vi "Display Required Helper.vi"(8 "Display Required Argument":T2, 11 "Module Data":T3) -> (0 "Display Required (Reply Payload)":T1, 1 "Message":string, 3 "Module Data out":T3)   [LabVIEW 2024, in "DQMH Power Requests.lvlib"]
doc: "<b>Note:</b> This VI was modified by the <b>Validate DQMH Module</b> tool to turn off automatic error handling.\n\n<b>Note:</b> This VI was modified by the <b>Validate DQMH Module</b> tool to be shared clone reentrant."
uses:
  DQMH Power Requests.lvlib
  Module Data--cluster.ctl
  Display Required Argument--cluster.ctl
  Display Required (Reply Payload)--cluster.ctl
  Power-Requests/Power Availabilty Requests/Type Defs/Power Availiability Requests Functions.ctl
  Power-Requests/Power Availabilty Requests/Type Defs/Power Request Type.ctl
  <vilib>/Utility/error.llb/Error Cluster From Error Code.vi
  <vilib>/ErrorRing/Error Ring.xnode
  Power-Requests/Power Requests.lvlib
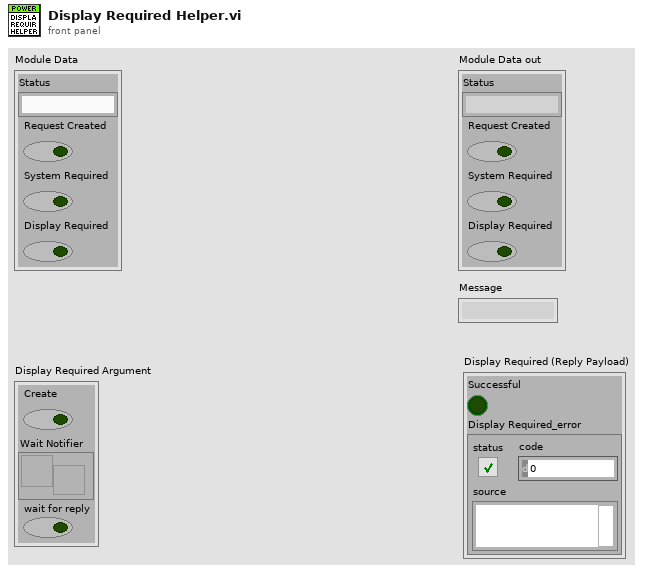
[diagram p1: front panel]
types:
  T1 = typedef "DQMH Power Requests.lvlib/Display Required (Reply Payload)--cluster.ctl" = cluster{"Successful":bool, "Display Required_error":errorcluster}
  T2 = typedef "DQMH Power Requests.lvlib/Display Required Argument--cluster.ctl" = cluster{"Create":bool, "Wait Notifier":refnum<notifier>, "wait for reply":bool}
  T3 = typedef "DQMH Power Requests.lvlib/Module Data--cluster.ctl" = cluster{"Status":string, "Request Created":bool, "System Required":bool, "Display Required":bool}
  T4 = typedef "Power Requests.lvlib/Power Request Type.ctl" = enum32{"Power Request Display Required", "Power Request System Required", "Power Request Away Mode Required", "Power Request Execution Required"}
  T5 = typedef "Power Requests.lvlib/Power Availiability Requests Functions.ctl" = enum32{"Power Create Request", "Power Set Request", "Power Clear Request", "Close Handle"}
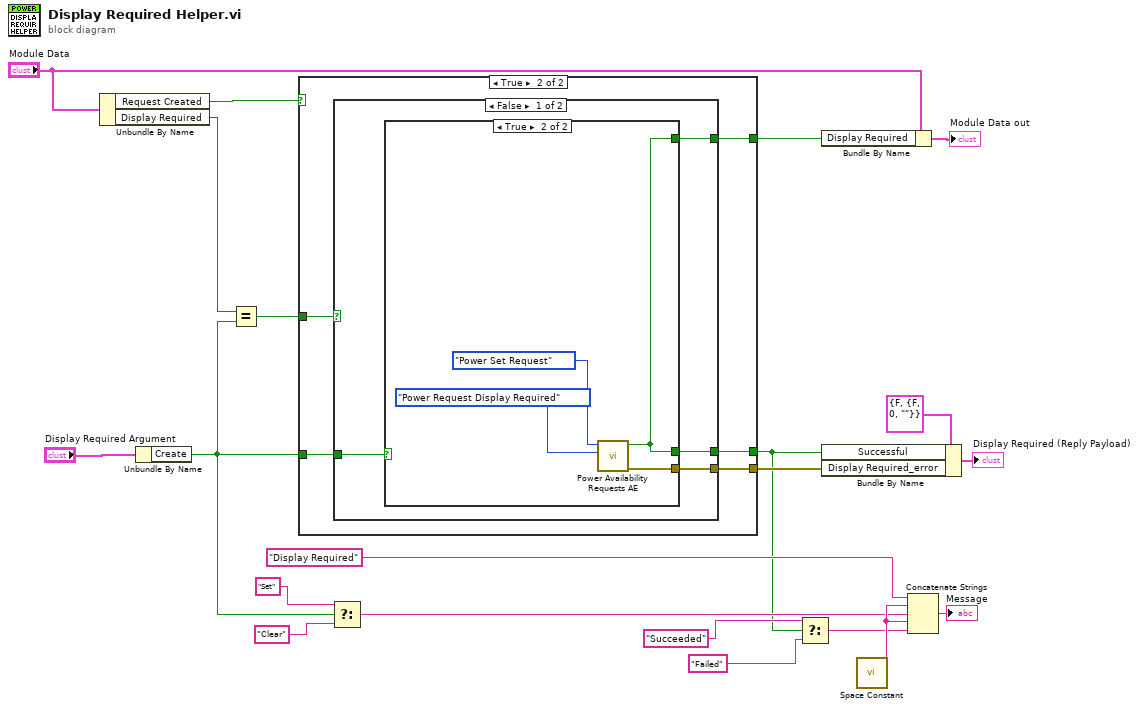
[diagram p0: block diagram]
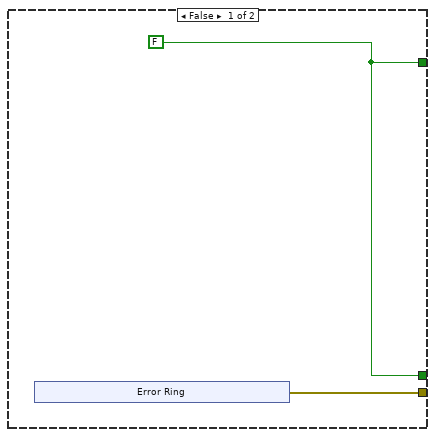
[diagram p2: hidden frame]
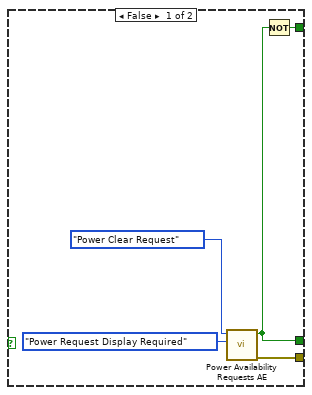
[diagram p3: hidden frame]
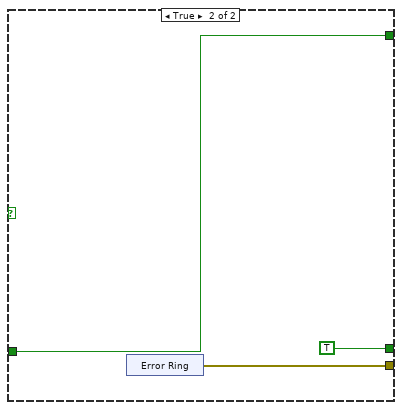
[diagram p4: hidden frame]
diagram:
  n1 = Unbundle By Name("Module Data") -> ("Request Created"=w15:bool, "Display Required"=w13:bool)
  n2 = Unbundle By Name("Display Required Argument") -> ("Create"=w1:bool)
  n3 = Equal?(x=w13, y=w1) -> (x = y?=w12:bool)
  n4 = case shown="True" w15 {
    tunnel: [w23 w31] -> w16
    tunnel: [w23 w29] -> w2
    tunnel: [w22 w28] -> w17
    tunnel: w12 -> [_ w32]
    tunnel: w1 -> [_ w30]
    frame False {
      w23 = FALSE
      n5 = xnode "Error Ring"() -> ("error out"=w22:errorcluster)
    }
    frame True {
      n6 = case shown="False" w32 {
        tunnel: [w33 w48] -> w31
        tunnel: w30 -> [w36 w48]
        tunnel: [w34 TRUE] -> w29
        tunnel: [w35 w46] -> w28
        frame False {
          n7 = case shown="True" w36 {
            tunnel: [w41 w45] -> w35
            tunnel: [w38 w44] -> w34
            tunnel: [w37 w44] -> w33
            frame False {
              n8 = call "Power Availability Requests AE.vi"("Power Request Type"=Power_Request_Type."Power Request Display Required", "Power Availability Requests Functions"=Power_Availiability_Requests_Functions."Power Clear Request") -> ("error out"=w41:errorcluster, "Success?"=w38:bool)  [unwired: 8 in]
              n9 = Not(x=w38) -> (.not. x?=w37:bool)
            }
            frame True {
              n10 = call "Power Availability Requests AE.vi"("Power Request Type"=Power_Request_Type."Power Request Display Required", "Power Availability Requests Functions"=Power_Availiability_Requests_Functions."Power Set Request") -> ("error out"=w45:errorcluster, "Success?"=w44:bool)  [unwired: 8 in]
            }
          }
        }
        frame True {
          n11 = xnode "Error Ring"() -> ("error out"=w46:errorcluster)
        }
      }
    }
  }
  n12 = Select(t="Set", s=w1, f="Clear") -> (s? t:f=w6:string)
  n13 = Select(t="Succeeded", s=w2, f="Failed") -> (s? t:f=w5:string)
  n14 = Bundle By Name(cluster="Module Data", "Display Required"=w16) -> (→"Module Data out":T3)
  n15 = Bundle By Name(cluster=T1 {"Successful"=FALSE, "Display Required_error"={"status"=FALSE, "code"=0, "source"=""}} ("Display Required (Reply Payload)"), "Successful"=w2, "Display Required_error"=w17) -> (→"Display Required (Reply Payload)":T1)
  n16 = call <vilib>:"Space Constant.vi"() -> ("String"=w9:string)
  n17 = Concatenate Strings("Display Required", w9, w6, w9, w5) -> (→"Message":string)
